vi "Load Configuration Settings from XML.vi"(8 "error in (no error)":errorcluster, 11 "User Specified":T1={"Vacuum Graph config"={"Log/Lin"=FALSE, "Show Backing"=FALSE, "Show Chamber"=FALSE}, "Hardware Configuration"={"VGC50"={"serial settings"={"port"="", "baud rate"=115200}, "device information"={"type"="", "model number"="", "serial number"="", "firmware version"="", "hardware version"=""}, "VGC"=refnum, "Backing SP"={"mode"=0, "thresholds"={"lower"=0.0, "upper"=0.0}, "on"=FALSE}, "Chamber SP"={"mode"=1, "thresholds"={"lower"=0.0, "upper"=0.0}, "on"=FALSE}}, "PTC10"={"serial settings"={"port"="GPIB0::22::INSTR", "baud rate"=115200}, "PTC10 Info"={"Manufacturer"="", "Instrument"="", "Serial Number"="", "Firmware"=""}, "VISA resource name"="", "pwmloop"="define pwmloop(#t=0 while (1) {waitforsample if(#pwm=0){relays=0}else{if(#t<#pwm) {relays=1}else{relays=3}}#t+=1 if  (#t>99){#t=0} pause 0.2 s})", "onecycle"="define onecycle (pwm=100 run pwmloop 5A.PID.Setpoint=-130.0 5A.PID.input=3C while(#3C>-129.0){pause 0.2 s}pwm=-130 pause 10 min pwm=0  5A.PID.SetPoint=50.0 while(#3C<49.0){pause 0.2 s} pause 10 min kill pwmloop)", "control"="define control (#count=1 while (#count>=0) {onecycle pause 1 s #count-=1})", "HeatDrive"="define Failsafe (while(1) {if (#Check <-20){relays=0 outputEnable Off}else{if(#Check>20){relays=0 outputEnable Off}} pause 1 s})", "ToAmbient"="define ToAmbient(if(#3C>25.0){pwm=100 run pwmloop while(#3C>#25.0){pause 0.5 s} pwm=0 kill pwmloop}else{#5A.PID.setpoint=20.0 while(#3C<15.0){pause 0.5 s} outputenable off})", "StartupCode"="system.display.Monitors Show", "LogChannels"=[], "Heater O/P Channel"="", " Control Input"="", "TAmbient"=20.0, "AmbientTolerance"=5.0, "PID Params"={"P"=1.14, "I"=0.012, "D"=21.68, "Set"=0.0}, "TestCycleParameters"={"TAmb"=20.0, "HeaterTestTemp"=20.0, "HeaterTestDwell(min)"=1, "HeaterTestDuration"=1, "MinOpTemp"=-131.5, "MinOpDwell(min)"=30, "TestHeatingRate (deg/min)"=0.4, "SurviveCycleParameters"={"MinSurviveTemp"=-131.5, "MinSurvive Dwell(min)"=10, "MaxSurviveTemp"=50.0, "MaxSurviveDwell(min)"=30, "ControlInput"=2, "ColdStandOff"=4.0, "HotStandoff"=5.0, "SteadyPWM"=20, "MaxCoolingRate (deg/min)"=3.75, "MaxHeatingRate (deg/min)"=2.5}, "CycleType"=0, "MaxOpTemp"=-50.0, "MaxOpDwell(min)"=30}}}} {"Hardware Configuration"."PTC10"."TestCycleParameters"."CycleType" items=["Survival", "Operational"]; "Hardware Configuration"."PTC10"."TestCycleParameters"."SurviveCycleParameters"."SteadyPWM" min=0 max=100 step=1; "Hardware Configuration"."PTC10"."TestCycleParameters"."SurviveCycleParameters"."ControlInput" items=["3A", "3B", "3C", "3D", "4A", "4B", "4C", "4D"]; "Hardware Configuration"."PTC10"."PID Params"."D" min=0.0; "Hardware Configuration"."PTC10"."PID Params"."I" min=0.0; "Hardware Configuration"."PTC10"."PID Params"."P" min=0.0; "Hardware Configuration"."PTC10"."TAmbient" min=0.0 max=30.0; "Hardware Configuration"."PTC10"."serial settings"."baud rate" items=["9600"=9600, "19200"=19200, "38400"=38400, "57600"=57600, "115200"=115200]; "Hardware Configuration"."VGC50"."Chamber SP"."thresholds"."upper" format="%#_5p"; "Hardware Configuration"."VGC50"."Chamber SP"."thresholds"."lower" format="%#_5p"; "Hardware Configuration"."VGC50"."Chamber SP"."mode" items=["off", "on", "channel 1", "channel 2", "channel 3"]; "Hardware Configuration"."VGC50"."Backing SP"."thresholds"."upper" format="%#_5p"; "Hardware Configuration"."VGC50"."Backing SP"."thresholds"."lower" format="%#_5p"; "Hardware Configuration"."VGC50"."Backing SP"."mode" items=["off", "on", "channel 1", "channel 2", "channel 3"]; "Hardware Configuration"."VGC50"."serial settings"."baud rate" items=["9600"=9600, "19200"=19200, "38400"=38400, "57600"=57600, "115200"=115200]}) -> (0 "error out":errorcluster, 3 "User Specified Out":T1={"Vacuum Graph config"={"Log/Lin"=FALSE, "Show Backing"=FALSE, "Show Chamber"=FALSE}, "Hardware Configuration"={"VGC50"={"serial settings"={"port"="Inficon_VGC503", "baud rate"=115200}, "device information"={"type"="VGC503", "model number"="398-483", "serial number"="7433", "firmware version"="1.07", "hardware version"="1.0"}, "VGC"=refnum, "Backing SP"={"mode"=2, "thresholds"={"lower"=1.0, "upper"=5.0}, "on"=TRUE}, "Chamber SP"={"mode"=3, "thresholds"={"lower"=0.0001, "upper"=0.0005}, "on"=TRUE}}, "PTC10"={"serial settings"={"port"="Stanford_PTC10", "baud rate"=9600}, "PTC10 Info"={"Manufacturer"="Stanford Research Systems", "Instrument"=" PTC10 Programmable Temperature Controller", "Serial Number"=" 153826", "Firmware"=" version 4.56"}, "VISA resource name"="Stanford_PTC10", "pwmloop"="define pwmloop(#t=0 while (1) {waitforsample if(#pwm=0){relays=0}else{if(#t<#pwm) {relays=1}else{relays=3}}#t+=1 if  (#t>99){#t=0} pause 0.2 s})", "onecycle"="define onecycle (pwm=100 run pwmloop 5A.PID.Setpoint=-131.5 5A.PID.input=4D while(#4D>-130.5){pause 0.2 s}pwm=20 pause 20 min pwm=0  5A.PID.SetPoint=51.5 while(#4D<50.5){pause 0.2 s} pause 20 min kill pwmloop)", "control"="define control (while (#Cycles>0) {onecycle pause 1 s #Cycles-=1})", "HeatDrive"="define Failsafe (while(1) {if (#Check<-20){relays=0 outputEnable Off}else{if(#Check>20){relays=0 outputEnable Off}} pause 1 s})", "ToAmbient"="define ToAmbient(if(#3C>25.0){pwm=100 run pwmloop while(#3C>#25.0){pause 0.5 s} pwm=0 kill pwmloop}else{#5A.PID.setpoint=20.0 while(#3C<15.0){pause 0.5 s} outputenable off})", "StartupCode"="define ToAmbient(if(#3C>25.0){pwm=100 run pwmloop while(#3C>#25.0){pause 0.5 s} pwm=0 kill pwmloop}else{#5A.PID.setpoint=20.0 while(#3C<15.0){pause 0.5 s} outputenable off})", "LogChannels"=["Out 1", " I 1", " V 1", " R 1", " Out 2", " I 2", " V 2", " R 2", " PCB 2", " 3A", " 3B", " 3C", " 3D", " PCB 3", " 4A", " 4B", " 4C", " 4D", " PCB 4", " 5A", " 5B", " 5C", " 5D", " DIO", " Relays", " pwm", " Cycles", " Check"], "Heater O/P Channel"="", " Control Input"="", "TAmbient"=20.0, "AmbientTolerance"=5.0, "PID Params"={"P"=1.14, "I"=0.012, "D"=21.68, "Set"=0.0}, "TestCycleParameters"={"TAmb"=20.0, "HeaterTestTemp"=20.0, "HeaterTestDwell(min)"=1, "HeaterTestDuration"=1, "MinOpTemp"=-131.5, "MinOpDwell(min)"=30, "TestHeatingRate (deg/min)"=0.4, "SurviveCycleParameters"={"MinSurviveTemp"=-131.5, "MinSurvive Dwell(min)"=10, "MaxSurviveTemp"=50.0, "MaxSurviveDwell(min)"=30, "ControlInput"=2, "ColdStandOff"=4.0, "HotStandoff"=5.0, "SteadyPWM"=20, "MaxCoolingRate (deg/min)"=3.75, "MaxHeatingRate (deg/min)"=2.5}, "CycleType"=0, "MaxOpTemp"=-50.0, "MaxOpDwell(min)"=30}}}} {"Hardware Configuration"."PTC10"."TestCycleParameters"."CycleType" items=["Survival", "Operational"]; "Hardware Configuration"."PTC10"."TestCycleParameters"."SurviveCycleParameters"."SteadyPWM" min=0 max=100 step=1; "Hardware Configuration"."PTC10"."TestCycleParameters"."SurviveCycleParameters"."ControlInput" items=["3A", "3B", "3C", "3D", "4A", "4B", "4C", "4D"]; "Hardware Configuration"."PTC10"."PID Params"."D" min=0.0; "Hardware Configuration"."PTC10"."PID Params"."I" min=0.0; "Hardware Configuration"."PTC10"."PID Params"."P" min=0.0; "Hardware Configuration"."PTC10"."TAmbient" min=0.0 max=30.0; "Hardware Configuration"."PTC10"."serial settings"."baud rate" items=["9600"=9600, "19200"=19200, "38400"=38400, "57600"=57600, "115200"=115200]; "Hardware Configuration"."VGC50"."Chamber SP"."thresholds"."upper" format="%#_5p"; "Hardware Configuration"."VGC50"."Chamber SP"."thresholds"."lower" format="%#_5p"; "Hardware Configuration"."VGC50"."Chamber SP"."mode" items=["off", "on", "channel 1", "channel 2", "channel 3"]; "Hardware Configuration"."VGC50"."Backing SP"."thresholds"."upper" format="%#_5p"; "Hardware Configuration"."VGC50"."Backing SP"."thresholds"."lower" format="%#_5p"; "Hardware Configuration"."VGC50"."Backing SP"."mode" items=["off", "on", "channel 1", "channel 2", "channel 3"]; "Hardware Configuration"."VGC50"."serial settings"."baud rate" items=["9600"=9600, "19200"=19200, "38400"=38400, "57600"=57600, "115200"=115200]})   [LabVIEW 2024]
doc: "Attempts to load previous user specified settings from an XML file.\n\nThis VI will not generate an error. If a suitable XML file can't be loaded and parsed then it will simply return the default settings."
uses:
  controls/User Specified Data.ctl
  Program Files/National Instruments/LabVIEW 2024/instr.lib/PL Inficon VGC/PL Inficon VGC.lvclass
  controls/Vac Graph Config.ctl
  controls/HW Configuration.ctl
  controls/VGC50.ctl
  controls/SRS PTC10.ctl
  controls/PID Params.ctl
  controls/TestCycleParams.ctl
  controls/SurviveCycleParams.ctl
  controls/ControlInput.ctl
  <vilib>/Utility/xml.llb/Read From XML File(string).vi
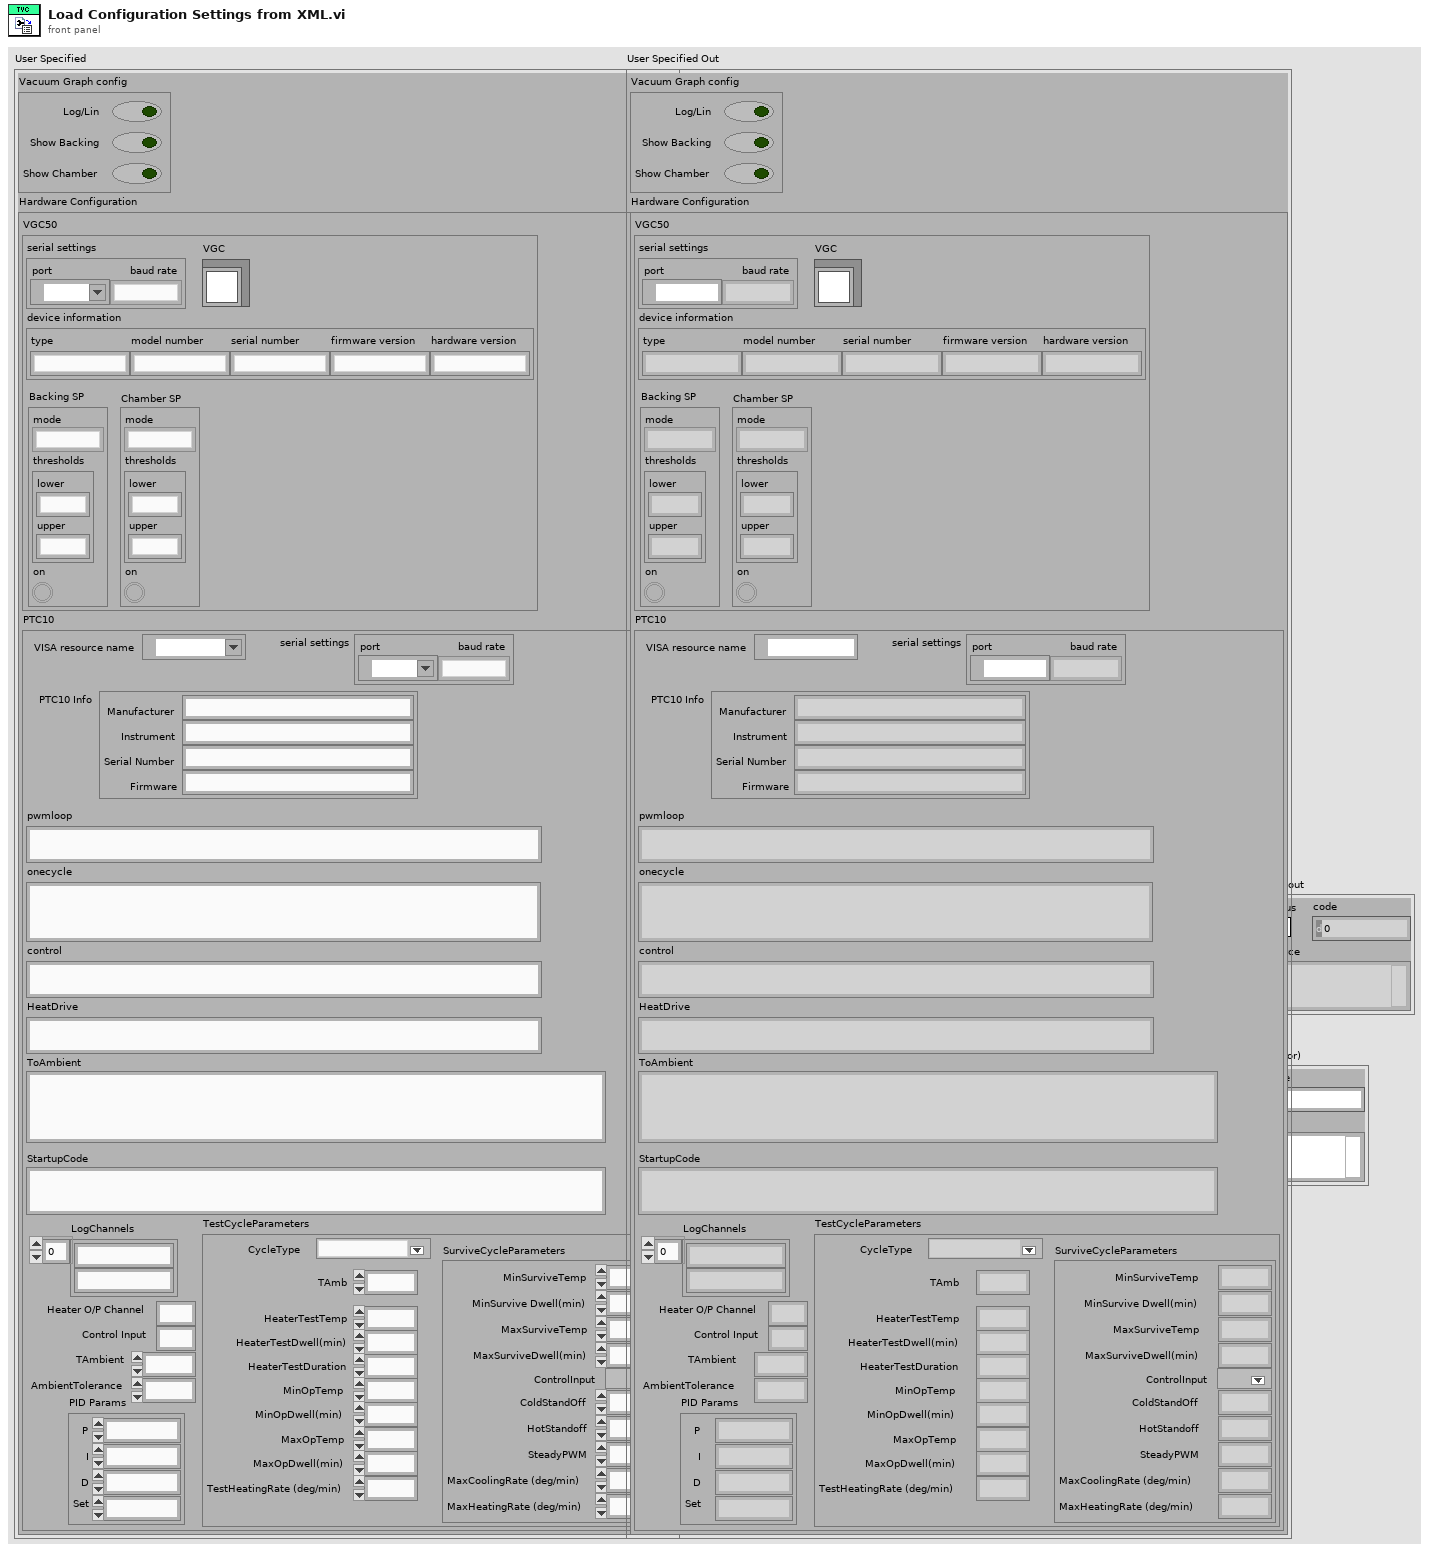
[diagram p1: front panel]
types:
  T1 = typedef "User Specified Data.ctl" = cluster{"Vacuum Graph config":T2, "Hardware Configuration":T3}
  T2 = typedef "Vac Graph Config.ctl" = cluster{"Log/Lin":bool, "Show Backing":bool, "Show Chamber":bool}
  T3 = typedef "HW Configuration.ctl" = cluster{"VGC50":T4, "PTC10":T5}
  T4 = typedef "VGC50.ctl" = cluster{"serial settings":cluster{"port":refnum<visa-resource-name>, "baud rate":u32}, "device information":cluster{"type":string, "model number":string, "serial number":string, "firmware version":string, "hardware version":string}, "VGC":refnum<class "PL Inficon VGC.lvclass">, "Backing SP":cluster{"mode":u16, "thresholds":cluster{"lower":dbl, "upper":dbl}, "on":bool}, "Chamber SP":cluster{"mode":u16, "thresholds":cluster{"lower":dbl, "upper":dbl}, "on":bool}}
  T5 = typedef "SRS PTC10.ctl" = cluster{"serial settings":cluster{"port":refnum<visa-resource-name>, "baud rate":u32}, "PTC10 Info":cluster{"Manufacturer":string, "Instrument":string, "Serial Number":string, "Firmware":string}, "VISA resource name":refnum<visa-resource-name>, "pwmloop":string, "onecycle":string, "control":string, "HeatDrive":string, "ToAmbient":string, "StartupCode":string, "LogChannels":string[], "Heater O/P Channel":string, " Control Input":string, "TAmbient":dbl, "AmbientTolerance":dbl, "PID Params":T6, "TestCycleParameters":T7}
  T6 = typedef "PID Params.ctl" = cluster{"P":dbl, "I":dbl, "D":dbl, "Set":dbl}
  T7 = typedef "TestCycleParams.ctl" = cluster{"TAmb":dbl, "HeaterTestTemp":dbl, "HeaterTestDwell(min)":i32, "HeaterTestDuration":i32, "MinOpTemp":dbl, "MinOpDwell(min)":i32, "TestHeatingRate (deg/min)":dbl, "SurviveCycleParameters":T8, "CycleType":u16, "MaxOpTemp":dbl, "MaxOpDwell(min)":i32}
  T8 = typedef "SurviveCycleParams.ctl" = cluster{"MinSurviveTemp":dbl, "MinSurvive Dwell(min)":i32, "MaxSurviveTemp":dbl, "MaxSurviveDwell(min)":i32, "ControlInput":T9, "ColdStandOff":dbl, "HotStandoff":dbl, "SteadyPWM":i32, "MaxCoolingRate (deg/min)":dbl, "MaxHeatingRate (deg/min)":dbl}
  T9 = typedef "ControlInput.ctl" = u16
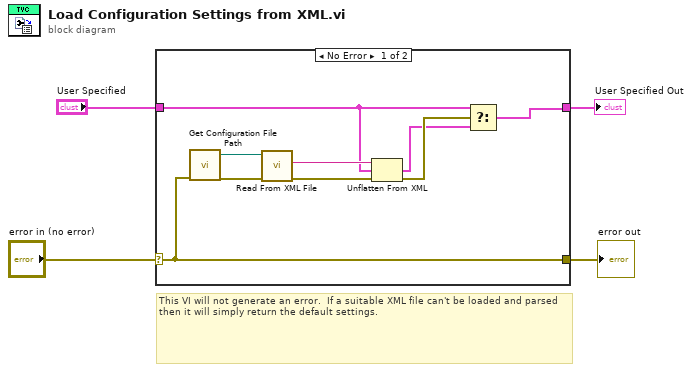
[diagram p0: block diagram]
diagram:
  # "This VI will not generate an error.  If a suitable XML file can't be loaded and parsed then it will simply return the default settings."
  n1 = case shown="No Error" "error in (no error)" {
    selector: "error in (no error)" -> [w10 w15]
    tunnel: [w10 w15] -> w3
    tunnel: "User Specified" -> [w7 w14]
    tunnel: [w5 w14] -> w1
    frame No Error {
      n2 = call "Get Configuration File Path.vi"("error in (no error)"=w10) -> ("error out"=w12:errorcluster, "XML File Path"=w13:path)  [unwired: 9 in]
      n3 = call-poly <vilib>:"Read From XML File.vi"("error in (no error)"=w12, "XML File Path"=w13) -> ("error out"=w9:errorcluster, "XML Elements"=w11:string)  [unwired: 7 in, 1 out]
      n4 = Unflatten From XML(xml string=w11, type=w7, error in (no error)=w9) -> (value=w6:T1, error out=w8:errorcluster)
      n5 = Select(t=w7, s=w8, f=w6) -> (s? t:f=w5:T1)
    }
    frame Error {
    }
  }
  "error out" <- w3
  "User Specified Out" <- w1
